vi "16Chennels_ExtraWindow.vi"(0 "Spectral Waveform":cluster{dbl[], dbl[]}(graph), 3 "Energy Data":dbl, 4 "New Energy":bool, 6 "Shot # in":string, 8 "Ch 16 Status":bool, 9 "Colors [4]":cluster{u32, u32}[](array[cluster])) -> ()   [LabVIEW 2020]
panel:
  out "Shot #":string
  out "5th Stage":dbl(graph)
  # "Energy"
  # "J"
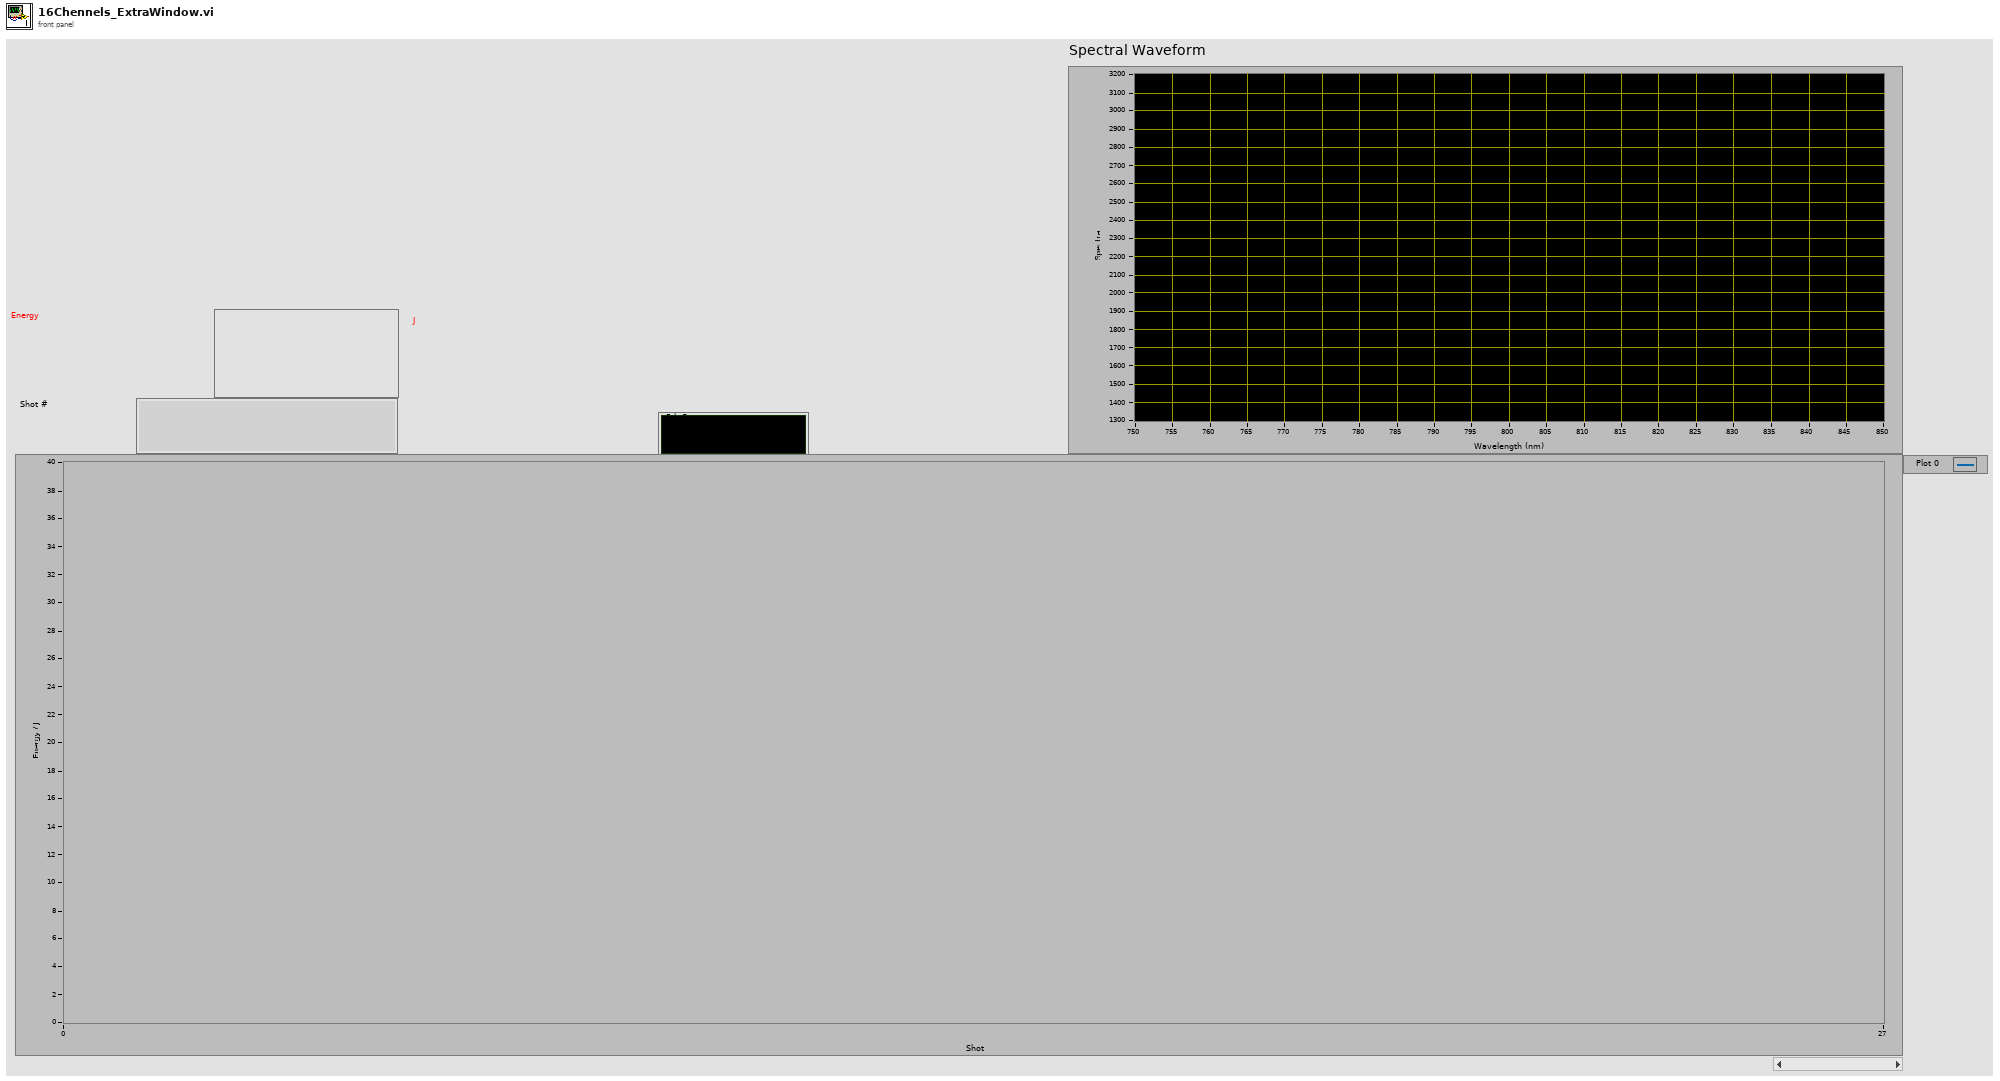
[diagram p1: front panel]
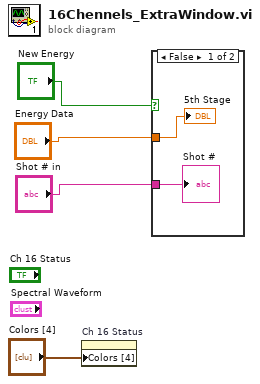
[diagram p0: block diagram]
diagram:
  n1 = property on="Ch 16 Status" class="Bool (strict)"("Colors [4]"="Colors [4]") -> ()  [unwired: 2 in, 2 out]
  n2 = case shown="False" "New Energy" {
    tunnel: "Energy Data" -> [w6 _]
    tunnel: "Shot # in" -> [w5 _]
    frame False {
      "5th Stage" <- w6
      "Shot #" <- w5
    }
    frame True {
    }
  }
